vi "Collect Param - Bool.vi"(8 "Error in":errorcluster caption="Error in (no error)", 9 "Value":bool, 10 "Param Name":string="user_field_names", 11 "Params Array In":T1[](array[typedef])) -> (0 "Error out":errorcluster, 3 "Params Array Out":T1[](array[typedef]))   [LabVIEW 2018]
uses:
  TypeDef/Param.ctl
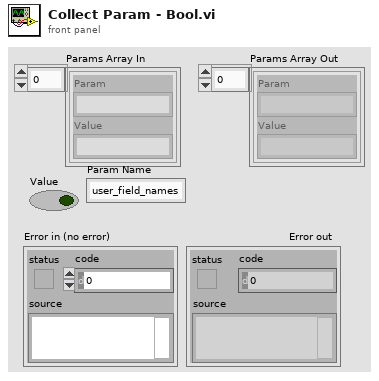
[diagram p1: front panel]
types:
  T1 = typedef "Param.ctl" = cluster{"Param":string, "Value":string}
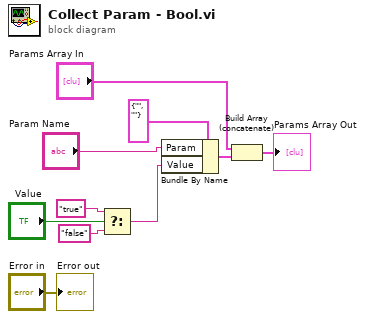
[diagram p0: block diagram]
diagram:
  n1 = Select(t="true", s="Value", f="false") -> (s? t:f=w9:string)
  n2 = Bundle By Name(cluster=T1 {"Param"="", "Value"=""} ("Cluster"), "Param"="Param Name", "Value"=w9) -> (w3:T1)
  n3 = Build Array (concatenate)("Params Array In", w3) -> (→"Params Array Out":T1[])
  "Error out" <- "Error in"
